vi "Limit URI.vi"(8 "error in":errorcluster, 11 "base path":path) -> (0 "error out":errorcluster)   [LabVIEW 2014]
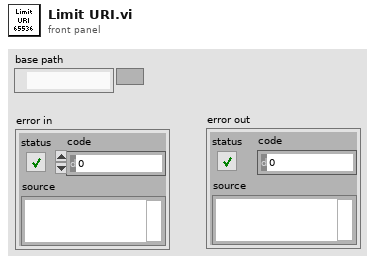
[diagram p1: front panel]
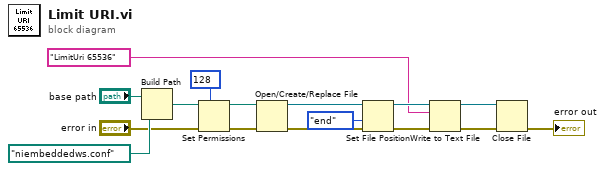
[diagram p0: block diagram]
diagram:
  n1 = Build Path(base path="base path", name or relative path=path "niembeddedws.conf") -> (appended path=w9:path)
  n2 = Set Permissions(7:i16 128 ("permissions"), 8:"error in", 11:w9) -> (0:w1:errorcluster, 3:w6:path)  [unwired: 2 in]
  n3 = Open/Create/Replace File(file path (use dialog)=w6, error in=w1) -> (refnum out=w16:refnum<file>, error out=w15:errorcluster)  [unwired: 4 in, 1 out]
  n4 = Set File Position(refnum=w16, from (0:start)=enum16{"start", "end", "current"}."end", error in=w15) -> (refnum out=w14:refnum<file>, error out=w13:errorcluster)  [unwired: 1 in]
  n5 = Write to Text File(file (use dialog)=w14, text="LimitUri 65536", error in=w13) -> (refnum out=w12:refnum<file>, error out=w11:errorcluster)  [unwired: 1 in, 1 out]
  n6 = Close File(refnum=w12, error in=w11) -> (error out=→"error out":errorcluster)  [unwired: 1 out]
